vi "CRYDisplay.vi"(0 "Setup in":T1={"No.VI"=0, "Category"="", "StepName"="", "Seq setup flattened"="", "Comment"="", "Steps config."=[], "Jump config"=[], "Start"=0.0, "Increment"=0.0, "Name"="Pa", "Unit"="Pa", "Y data"=1, "Y prefix"="", "Y dB ref"=1.0, "Y unit"="", "Repeat State Array"=[]} {"Repeat State Array"."Start" format="%#_5g"; "Y dB ref" format="%.1f"; "Y data" items=["dB", "Lin"]; "Start" format="%#_5g"}, 5 "Data in":T5 {"Z data" items=["dB", "Lin"]; "X data" items=["dB", "Lin"]; "Y data" items=["dB", "Lin"]; "Z dB ref" format="%.1f"; "Z axis" items=["Log", "Lin"]; "X dB ref" format="%.1f"; "X axis" items=["Log", "Lin"]; "Y axis" items=["Log", "Lin"]; "Y dB ref" format="%.1f"; "Curve"."z" format="%.2f"; "Curve"."y" format="%.2f"; "Curve"."x" format="%.2f"}, 7 "Results in":T3 {"Margin" format="%.2f"}, 9 "Seq Setup in":string, 11 "Step name":string, 12 "Hardware in":string, 13 "Calibration in":string) -> (3 "Types Out":string[](array[string]), 4 "Inserted Names Out":string[](array[string]), 6 "Data out":T5 {"Z data" items=["dB", "Lin"]; "X data" items=["dB", "Lin"]; "Y data" items=["dB", "Lin"]; "Z dB ref" format="%.1f"; "Z axis" items=["Log", "Lin"]; "X dB ref" format="%.1f"; "X axis" items=["Log", "Lin"]; "Y axis" items=["Log", "Lin"]; "Y dB ref" format="%.1f"; "Curve"."z" format="%.2f"; "Curve"."y" format="%.2f"; "Curve"."x" format="%.2f"}, 8 "Results out":T3 {"Margin" format="%.2f"}, 10 "Wave out":T2[](array[typedef]) {"Y dB ref" format="%.1f"; "Y axis" items=["Log", "Lin"]; "Y data" items=["dB", "Lin"]; "X data" items=["dB", "Lin"]})   [LabVIEW 2013]
uses:
  Typedef Control/CRYData Cluster Array.ctl
  Typedef Control/CRYData Cluster.ctl
  Typedef Control/CRYResult Cluster Array.ctl
  Typedef Control/CRYResult Cluster.ctl
  Typedef Control/CRYWaveform Cluster.ctl
  Typedef Control/CRYStep.ctl
  Calibration/SubVI/CRYCal Global.vi
  CRYProject/CRYProject Editor Global.vi
  CRYWindow/DataView/VIEW/CRYView Global.vi
panel:
  # "Display run"
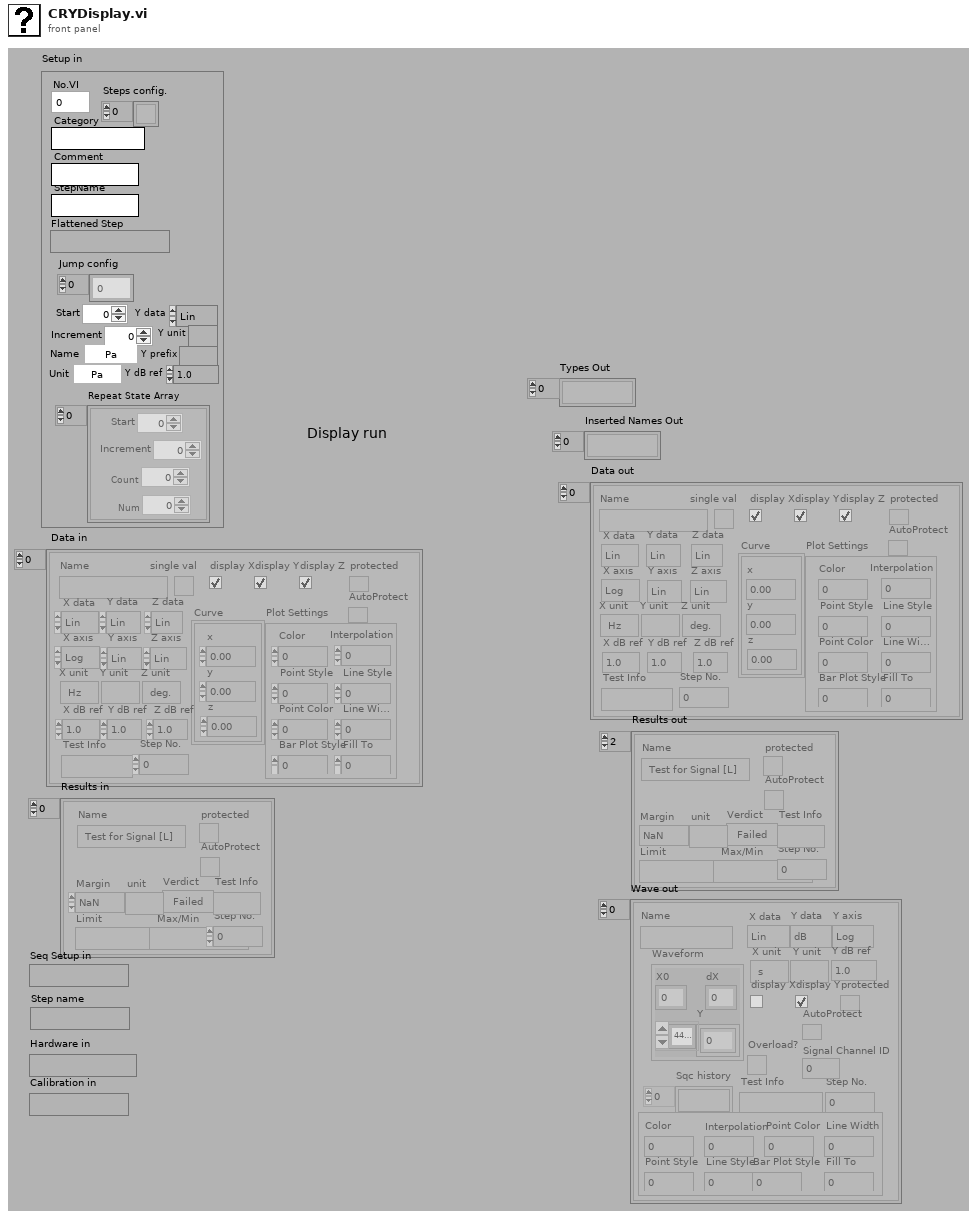
[diagram p1: front panel]
types:
  T1 = typedef "CRYStep.ctl" = cluster{"No.VI":i32, "Category":string, "StepName":string, "Seq setup flattened":string, "Comment":string, "Steps config.":bool[], "Jump config":i32[], "Start":dbl, "Increment":dbl, "Name":string, "Unit":string, "Y data":u16, "Y prefix":string, "Y dB ref":dbl, "Y unit":string, "Repeat State Array":cluster{"Start":dbl, "Increment":dbl, "Count":i32, "Num":i32}[]}
  T2 = typedef "CRYWaveform Cluster.ctl" = cluster{"Waveform":cluster{"X0":dbl, "dX":dbl, "Y":sgl[]}, "X data":u16, "Y data":u16, "Y axis":u16, "X unit":string, "Y unit":string, "Y dB ref":dbl, "display Y":bool, "display X":bool, "Overload?":bool, "Test Info":string, "Step No.":i32, "Name":string, "protected":bool, "Sqc history":string[], "Signal Channel ID":i32, "Plot Settings":cluster{"Color":u32, "Interpolation":u8, "Point Style":u8, "Line Style":u8, "Point Color":u32, "Line Width":u8, "Bar Plot Style":u8, "Fill To":i16}, "AutoProtect":bool}
  T3 = typedef "CRYResult Cluster Array.ctl" = T4[]
  T4 = typedef "CRYResult Cluster.ctl" = cluster{"Name":string, "Margin":dbl, "unit":string, "Verdict":bool, "Limit":string, "Max/Min":string, "protected":bool, "Step No.":i32, "Test Info":string, "AutoProtect":bool}
  T5 = typedef "CRYData Cluster Array.ctl" = T6[]
  T6 = typedef "CRYData Cluster.ctl" = cluster{"Name":string, "Curve":cluster{"x":dbl, "y":dbl, "z":dbl}[], "X data":u16, "Y data":u16, "Z data":u16, "X axis":u16, "Y axis":u16, "Z axis":u16, "X unit":string, "Y unit":string, "Z unit":string, "X dB ref":dbl, "Y dB ref":dbl, "Z dB ref":dbl, "single val":bool, "protected":bool, "display X":bool, "display Y":bool, "display Z":bool, "Test Info":string, "Step No.":i32, "Plot Settings":cluster{"Color":u32, "Interpolation":u8, "Point Style":u8, "Line Style":u8, "Point Color":u32, "Line Width":u8, "Bar Plot Style":u8, "Fill To":i16}, "AutoProtect":bool}
  T7 = typedef "CRYGraph Property.ctl" = cluster{"LegendShow":bool, "Legend Splitter Position":dbl, "Data Names":string[], "Item Symbols":i32[], "Color Array":u32[], "Flattened Plot Property":string, "CursorShow":bool, "Flattened Cursor Property":string, "Graph Number":i32, "Flattened Scale Property":string, "PreviewShow":bool, "MagnitudeShow":bool, "PaletteShow":bool, "XYShow":bool, "FrequencyShow":bool, "Frequency Splitter Position":dbl, "XYGraph Splitter Position":dbl, "Frequency Symbols":i32[], "LegendVScrollShow":bool, "FrequencyVScrollShow":bool, "PhaseShow":bool, "Title Name":string}
  T8 = cluster{"EventName":string, "Arg1":string, "Numeric":u16, "Numeric 2":u16, "AddSteps ":refnum<vi>, "Arg1 2":string, "Arg1 3":string, "Boolean":bool}
  T9 = cluster{"sAction":string, "sType":string, "sQueueName":string, "sGraphName":string, "sData":string, "nData":i32, "pVIRef":refnum<vi>, "pSPRef":refnum<vi>}
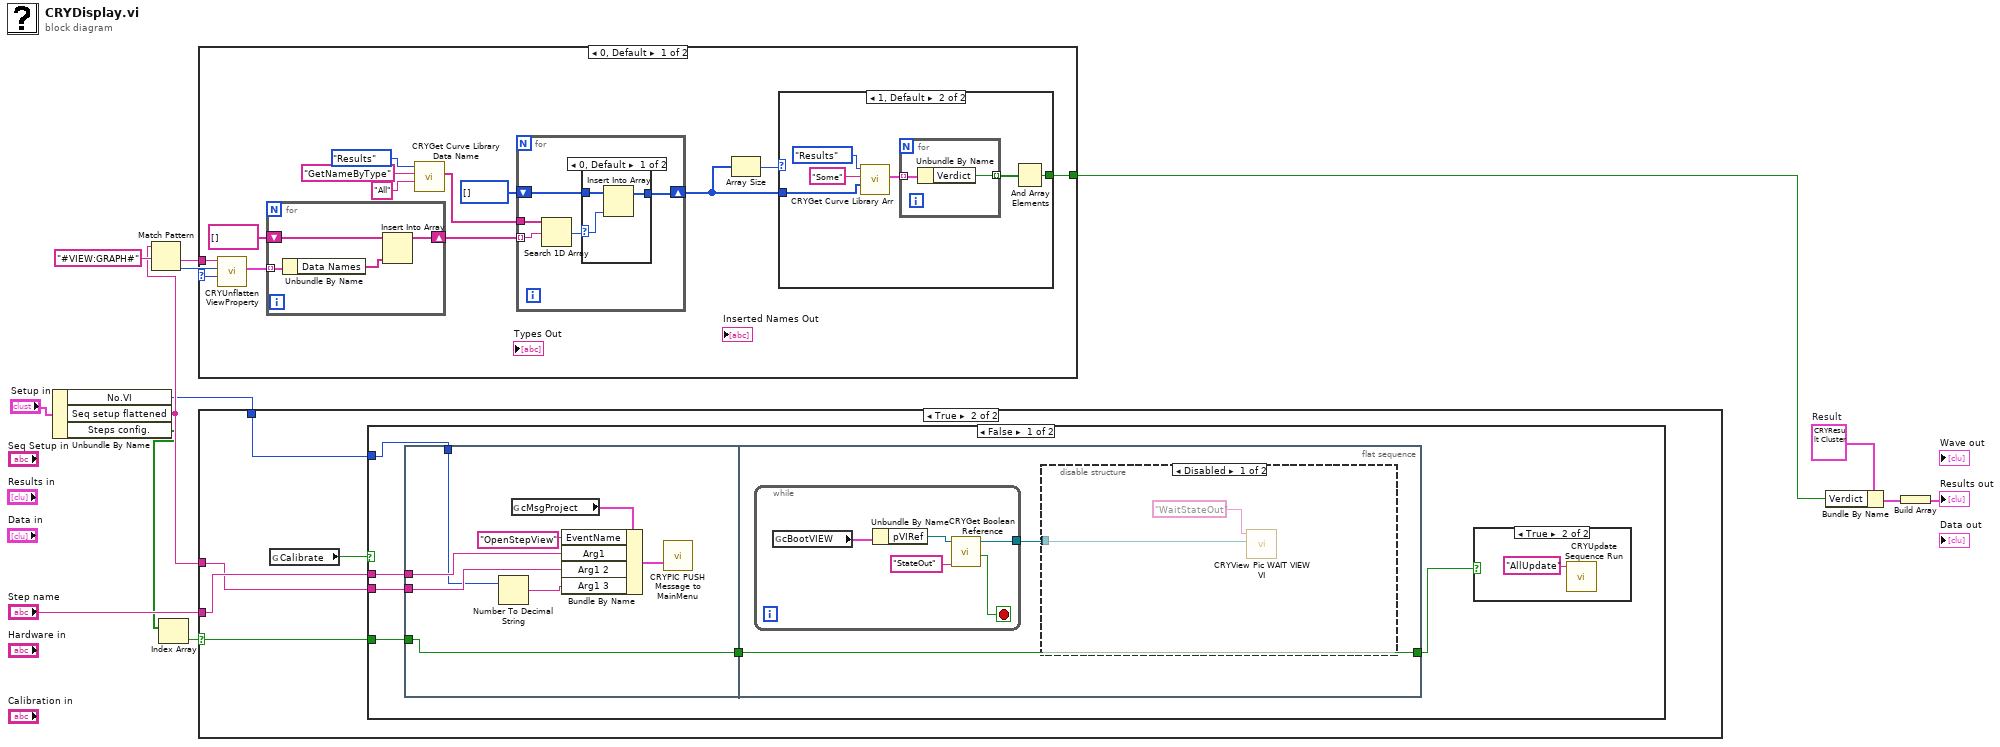
[diagram p0: block diagram]
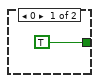
[diagram p2: hidden frame]
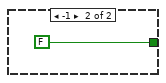
[diagram p4: hidden frame]
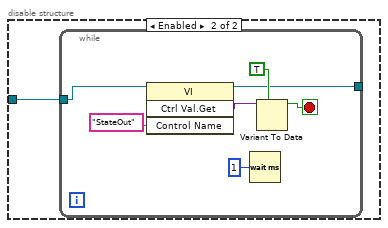
[diagram p7: hidden frame]
diagram:
  w8 = T4 {"Name"="Test for Signal [L]", "Margin"=nan, "unit"="", "Verdict"=FALSE, "Limit"="", "Max/Min"="", "protected"=FALSE, "Step No."=0, "Test Info"="", "AutoProtect"=FALSE}  # Result
  n1 = Unbundle By Name("Setup in") -> ("No.VI"=w1:i32, "Seq setup flattened"=w4:string, "Steps config."=w3:bool[])
  n2 = Match Pattern(string=w4, regular expression="#VIEW:GRAPH#") -> (after substring=w9:string, offset past match=w10:i32)  [unwired: 1 in, 2 out]
  n3 = Index Array(array=w3) -> (element=w12:bool)  [unwired: 1 in]
  n4 = case shown="0, Default" w10 {
    tunnel: w9 -> [w25 _]
    tunnel: [w16 FALSE] -> w2
    frame 0, Default {
      n5 = call "CRYUnflatten ViewProperty.vi"("Flatten ViewPro"=w25) -> ("ViewPro Cluster"=w24:T7[])  [unwired: 8 in, 2 out]
      n6 = for {
        tunnel: w24 -> [w47] mode=indexing
        shift-right: [w44] -> w19
        shift-left: string[] [] ("Data Names") -> [w46]
        n7 = Unbundle By Name(w47) -> ("Data Names"=w45:string[])
        n8 = Insert Into Array(array=w46, new element=w45) -> (w44:string[])  [unwired: 1 in]
      }
      n9 = call "CRYGet Curve Library Data Name.vi"("sOption"="All", "sAction"="GetNameByType", "Type"=enum16{"Curves", "Values", "Results", "WFM"}."Results") -> ("sNames"=w20:string[])  [unwired: 5 in, 3 out]
      n10 = for {
        tunnel: w20 -> [w39]
        tunnel: w19 -> [w38] mode=indexing
        shift-right: [w35] -> w15
        shift-left: i32[] [] -> [w36]
        n11 = Search 1D Array(1D array=w39, element=w38) -> (index of element=w37:i32)  [unwired: 1 in]
        n12 = case shown="0, Default" w37 {
          selector: w37 -> [w40 _]
          tunnel: [w42 w43] -> w35
          tunnel: w36 -> [w41 w43]
          frame 0, Default {
            n13 = Insert Into Array(array=w41, new element=w40) -> (w42:i32[])  [unwired: 1 in]
          }
          frame -1 {
          }
        }
      }
      n14 = Array Size(array=w15) -> (size(s)=w14:i32)
      n15 = case shown="1, Default" w14 {
        tunnel: [TRUE w29] -> w16
        tunnel: w15 -> [_ w27]
        frame 0 {
        }
        frame 1, Default {
          n16 = call "CRYGet Curve Library Arr.vi"("Index"=w27, "sOption"="Some", "Type In"=enum16{"Curves", "Values", "Results", "WFM"}."Results") -> ("Results"=w31:T3)  [unwired: 6 in, 2 out]
          n17 = for {
            tunnel: w31 -> [w34] mode=indexing
            tunnel: [w33] -> w30 mode=indexing
            n18 = Unbundle By Name(w34) -> ("Verdict"=w33:bool)
          }
          n19 = And Array Elements(Boolean array=w30) -> (logical AND=w29:bool)
        }
      }
    }
    frame -1 {
    }
  }
  n20 = case shown="True" w12 {
    selector: w12 -> [_ w51]
    tunnel: w4 -> [_ w52]
    tunnel: "Step name" -> [_ w53]
    tunnel: w1 -> [_ w50]
    frame False {
    }
    frame True {
      n21 = global read "CRYCal Global.vi" "Calibrate"() -> (w49:bool)
      n22 = case shown="False" w49 {
        tunnel: w53 -> [w59 _]
        tunnel: w52 -> [w58 _]
        tunnel: w51 -> [w57 _]
        tunnel: w50 -> [w55 _]
        frame False {
          n23 = flat-sequence {
            tunnel: w55 -> [w63]
            tunnel: w57 -> [w68]
            tunnel: w58 -> [w64]
            tunnel: w59 -> [w65]
            tunnel: [w68] -> w54
            tunnel: [w70] -> w56
            tunnel: w54 -> [w70]
            frame #0 {
              n24 = Number To Decimal String(number=w63) -> (decimal integer string=w62:string)  [unwired: 1 in]
              n25 = global read "CRYProject Editor Global.vi" "cMsgProject"() -> (w67:T8)
              n26 = Bundle By Name(cluster=w67, "EventName"="OpenStepView", "Arg1"=w65, "Arg1 2"=w64, "Arg1 3"=w62) -> (w61:T8)
              n27 = call "CRYPIC PUSH Message to MainMenu.vi"("cMsgProject"=w61) -> ()  [unwired: 11 in]
            }
            frame #1 {
              n28 = while {
                tunnel: [w81] -> w69
                stop <- w82 stop-if-true
                n29 = global read "CRYView Global.vi" "cBootVIEW"() -> (w85:T9)
                n30 = Unbundle By Name(w85) -> ("pVIRef"=w84:refnum<vi>)
                n31 = call "CRYGet Boolean Reference.vi"("Label Name"="StateOut", "VI Refnum"=w84) -> ("Exist?"=w82:bool, "VI Refnum Out"=w81:refnum<vi>)  [unwired: 7 in, 1 out]
              }
              n32 = disable-structure shown="Disabled" {
                disable-tunnel: w69 -> [w72 w73]
                frame Disabled {
                  n33 = call "CRYView Pic WAIT VIEW VI.vi"("vi reference"=w72, "sAction"="WaitStateOut") -> ()  [unwired: 9 in, 1 out]
                }
                frame Enabled {
                  n34 = while {
                    tunnel: [w75] -> _
                    tunnel: w73 -> [w74]
                    stop <- w77 stop-if-true
                    n35 = invoke class="VI" method="Ctrl Val.Get"(reference=w74, "Control Name"="StateOut") -> (reference out=w75:refnum<vi>, "Get Control Value Variant"=w79:variant)  [unwired: 2 in, 2 out]
                    n36 = Wait (ms)(milliseconds to wait=u32 1) -> ()  [unwired: 1 out]
                    n37 = Variant To Data(type=TRUE, Variant=w79) -> (data=w77:bool)  [unwired: 1 in, 1 out]
                  }
                }
              }
            }
          }
          n38 = case shown="True" w56 {
            frame False {
            }
            frame True {
              n39 = call "CRYUpdate Sequence Run.vi"("sOption"="AllUpdate") -> ()  [unwired: 11 in]
            }
          }
        }
        frame True {
        }
      }
    }
  }
  n40 = Bundle By Name(cluster=w8, "Verdict"=w2) -> (w7:T4)
  n41 = Build Array(w7) -> (→"Results out":T4[])
